vi "LV Image to Jpeg string (Quality).vi"(11 "JPEG File":path) -> (3 "Jpeg String":string)   [LabVIEW 2020]
uses:
  System.Drawing
panel:
  out "size":i32
  in  "Quality":u8=100
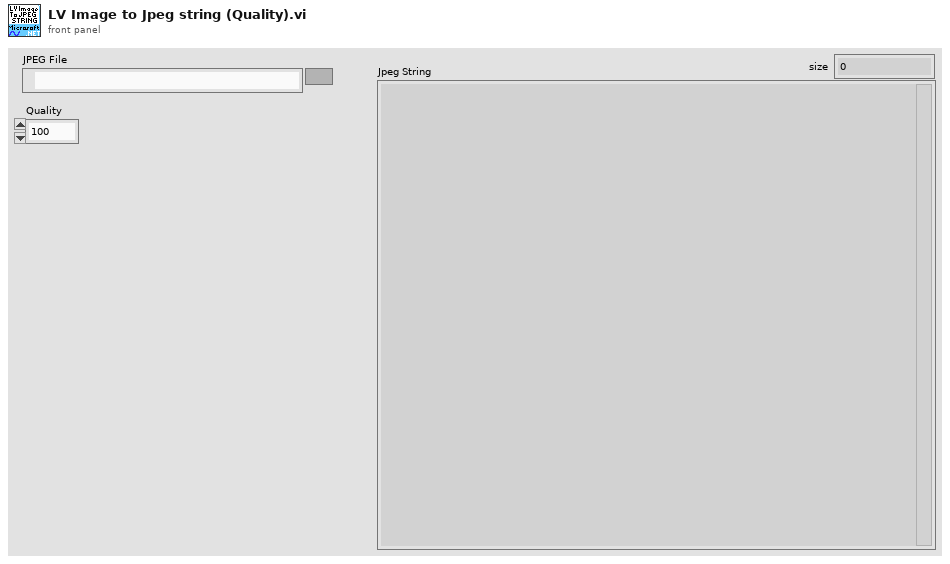
[diagram p1: front panel]
types:
  T1 = typedef "imagedata.ctl" = cluster{"image type":i32, "image depth":i32, "image":u8[], "mask":u8[], "colors":u32[], "Rectangle":cluster{"left":i16, "top":i16, "right":i16, "bottom":i16}}
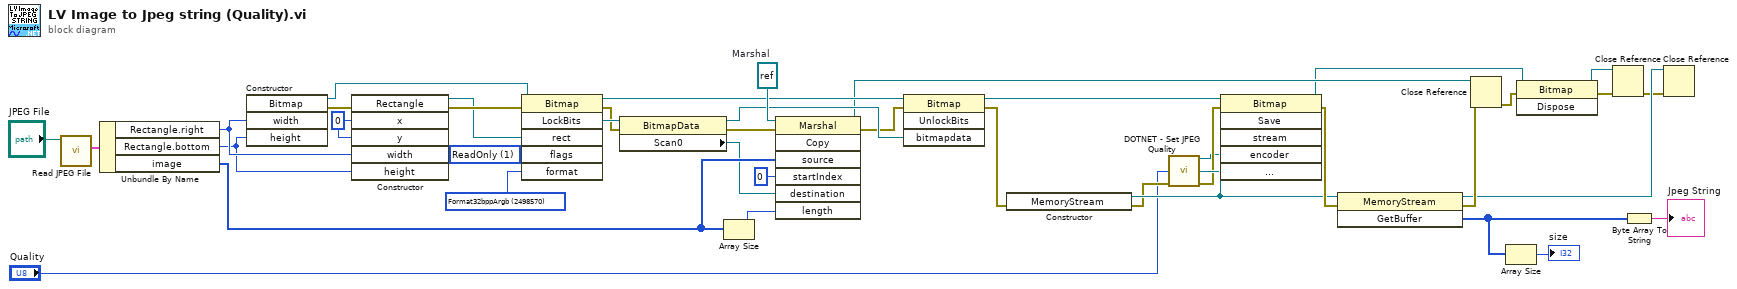
[diagram p0: block diagram]
diagram:
  w27 = refnum<k24> refnum  # Marshal
  w30 = 2498570 items=["DontCare, Undefined"=0, "Max"=15, "Indexed"=65536, "Gdi"=131072, "Format16bppRgb555"=135173, "Format16bppRgb565"=135174, "Format24bppRgb"=137224, "Format32bppRgb"=139273, "Format1bppIndexed"=196865, "Format4bppIndexed"=197634, "Format8bppIndexed"=198659, "Alpha"=262144, "Format16bppArgb1555"=397319, "PAlpha"=524288, "Format32bppPArgb"=925707, "Extended"=1048576, "Format16bppGrayScale"=1052676, "Format48bppRgb"=1060876, "Format64bppPArgb"=1851406, "Canonical"=2097152, "Format32bppArgb"=2498570, "Format64bppArgb"=3424269] ("format")
  w31 = 1 items=["ReadOnly"=1, "WriteOnly"=2, "ReadWrite"=3, "UserInputBuffer"=4] ("flags")
  w38 = 0 ("x")
  n1 = call <vilib>:"Read JPEG File.vi"("path to JPEG file"="JPEG File") -> ("image data"=w40:T1)  [unwired: 8 in, 2 out]
  n2 = Unbundle By Name(w40) -> ("Rectangle.right"=w37:i16, "Rectangle.bottom"=w36:i16, "image"=w24:u8[])
  n3 = constructor class="Bitmap"("width"=w37, "height"=w36) -> (reference out=w34:refnum<k24>, error out=w35:errorcluster)  [unwired: 3 in, 3 out]
  n4 = constructor class="Rectangle"(error in=w35, "x"=w38, "y"=w38, "width"=w37, "height"=w36) -> (reference out=w32:refnum<k24>, error out=w33:errorcluster)  [unwired: 2 in, 5 out]
  n5 = invoke class="Bitmap" method="LockBits"(reference=w34, error in=w33, "rect"=w32, "flags"=w31, "format"=w30) -> (reference out=w21:refnum<k24>, error out=w28:errorcluster, "LockBits"=w29:refnum<k24>)  [unwired: 1 in, 3 out]
  n6 = property class="BitmapData"(reference=w29, error in=w28) -> (reference out=w20:refnum<k24>, error out=w26:errorcluster, "Scan0"=w23:refnum<k24>)
  n7 = Array Size(array=w24) -> (size(s)=w22:i32)
  n8 = invoke class="Marshal" method="Copy"(reference=w27, error in=w26, "source"=w24, "startIndex"=0, "destination"=w23, "length"=w22) -> (reference out=w15:refnum<k24>, error out=w19:errorcluster)  [unwired: 1 in, 5 out]
  n9 = invoke class="Bitmap" method="UnlockBits"(reference=w21, error in=w19, "bitmapdata"=w20) -> (reference out=w18:refnum<k24>, error out=w17:errorcluster)  [unwired: 1 in, 2 out]
  n10 = constructor class="MemoryStream"(error in=w17) -> (reference out=w8:refnum<k24>, error out=w6:errorcluster)  [unwired: 2 in, 1 out]
  n11 = call "DOTNET - Set JPEG Quality.vi"("Quality"="Quality", "error in (no error)"=w6) -> ("ImageCodecInfo"=w3:refnum<k24>, "EncoderParameters"=w7:refnum<k24>, "error out"=w4:errorcluster)  [unwired: 11 in]
  n12 = invoke class="Bitmap" method="Save"(reference=w18, error in=w4, "stream"=w8, "encoder"=w3, "encoderParams"=w7) -> (reference out=w14:refnum<k24>, error out=w39:errorcluster)  [unwired: 1 in, 4 out]
  n13 = invoke class="MemoryStream" method="GetBuffer"(reference=w8, error in=w39) -> (reference out=w10:refnum<k24>, error out=w16:errorcluster, "GetBuffer"=w2:u8[])  [unwired: 1 in]
  n14 = Close Reference(reference=w15, error in (no error)=w16) -> (error out=w13:errorcluster)
  n15 = Array Size(array=w2) -> (size(s)=→"size":i32)
  n16 = invoke class="Bitmap" method="Dispose"(reference=w14, error in=w13) -> (reference out=w11:refnum<k24>, error out=w12:errorcluster)  [unwired: 1 in, 1 out]
  n17 = Close Reference(reference=w11, error in (no error)=w12) -> (error out=w9:errorcluster)
  n18 = Byte Array To String(unsigned byte array=w2) -> (string=→"Jpeg String":string)
  n19 = Close Reference(reference=w10, error in (no error)=w9) -> ()  [unwired: 1 out]
